vi "b2b2.vi"   [LabVIEW 2016, in "Moving Motor.lvrbt"]
uses:
  Moving Motor.lvrbt
  <vilib>/NXT/Block Support/NXT_InputPort.ctl
  <vilib>/NXT/Hardware/Plugins/Tetrix 180 deg Servo/Tetrix180ServoAddress.ctl
  <vilib>/NXT/Hardware/Plugins/Tetrix DC Motor/TetrixDCMotorAddress.ctl
  <vilib>/NXT/NXTIO Xnodes/NXTIONodeSubVIs/TETRIX IO Move Servos.vi
  <vilib>/NXT/NXTIO Xnodes/NXTIONodeSubVIs/TETRIX IO Move DC Motors.vi
  <vilib>/NXT/NXTIO Xnodes/NXTIONodeSubVIs/TETRIX IO Stop DC Motors.vi
  <vilib>/NXT/Dual Mode Library/Sensors/EV3_Ultrasonic_CM.vi
  <vilib>/NXT/Dual Mode Library/Waits/Wait_EV3_Ultrasonic_Centimeter_Closer.vi
  <vilib>/NXT/NXTIO Xnodes/AddressXNode/NXTIOAddress.xnode
  <vilib>/NXT/Subs/LVHSConnector.ctl
  <vilib>/NXT/NXTIO Xnodes/NXTIOXNode/NXTIO.xnode
  <vilib>/NXT/LegoClasses/BrickReference/BrickReference.lvclass
types:
  T1 = typedef "NXT_InputPort.ctl" = u32
  T2 = typedef "Tetrix180ServoAddress.ctl" = i32
  T3 = cluster{"Tetrix180Servo":T2, "Tetrix180Servo":T2}
  T4 = typedef "LVHSConnector.ctl" = refnum<class "BrickReference.lvclass">
  T5 = typedef "TetrixDCMotorAddress.ctl" = i32
  T6 = cluster{"TetrixDCMotor":T5, "TetrixDCMotor 2":T5}
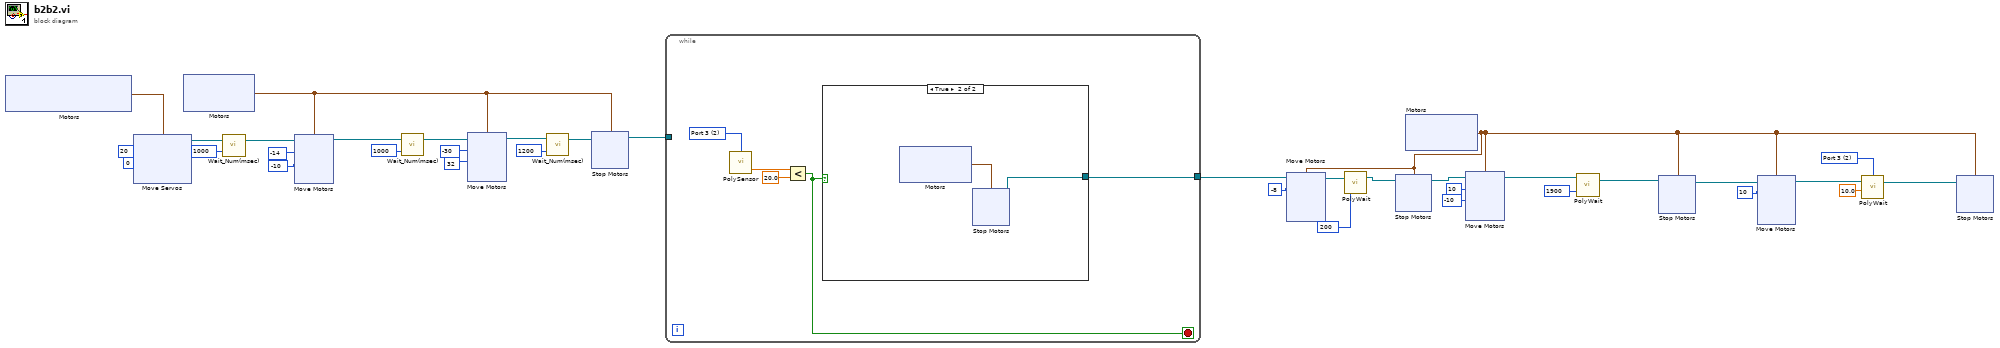
[diagram p0: block diagram]
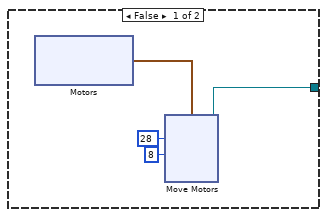
[diagram p2: hidden frame]
diagram:
  w7 = i8 -8 ("Power/Speed 1")
  w10 = T1 2 items=["Port 1", "Port 2", "Port 3", "Port 4"] ("Port (Port 1)")
  w12 = i8 10 ("Power/Speed 1")
  n1 = xnode "Motors"() -> ("Motor"=w35:T3)
  n2 = xnode "Move Servos"("Position 2"=u8 0, "Position 1"=u8 20, "Motors"=w35) -> ("NXT/EV3"=w32:T4)  [unwired: 1 in]
  n3 = xnode "Motors"() -> ("Motor"=w21:cluster{"TetrixDCMotor":T5, "TetrixDCMotor":T5})
  n4 = call <vilib>:"Wait_Num(msec).vi"("Time (100 msec)"=u32 1000, "NXT/EV3"=w32) -> ("NXT/EV3"=w31:T4)  [unwired: 2 in]
  n5 = xnode "Move Motors"("Power/Speed 2"=i8 -10, "Power/Speed 1"=i8 -14, "Motors"=w21, "NXT/EV3"=w31) -> ("NXT/EV3"=w27:T4)
  n6 = call <vilib>:"Wait_Num(msec).vi"("Time (100 msec)"=u32 1000, "NXT/EV3"=w27) -> ("NXT/EV3"=w20:T4)  [unwired: 2 in]
  n7 = xnode "Move Motors"("Power/Speed 2"=i8 32, "Power/Speed 1"=i8 -30, "Motors"=w21, "NXT/EV3"=w20) -> ("NXT/EV3"=w23:T4)
  n8 = call <vilib>:"Wait_Num(msec).vi"("Time (100 msec)"=u32 1200, "NXT/EV3"=w23) -> ("NXT/EV3"=w22:T4)  [unwired: 2 in]
  n9 = xnode "Stop Motors"("Motors"=w21, "NXT/EV3"=w22) -> ("NXT/EV3"=w19:T4)
  n10 = while {
    tunnel: w19 -> [_]
    tunnel: [w37] -> w6
    stop <- w38 stop-if-true
    w39 = T1 2 items=["Port 1", "Port 2", "Port 3", "Port 4"] ("Port (Port 1)")
    n11 = call-poly <vilib>:"PolySensor.vi"("Port (Port 1)"=w39) -> ("Centimeters"=w41:sgl)  [unwired: 2 in, 1 out]
    n12 = Less?(x=w41, y=sgl 20.0) -> (x < y?=w38:bool)
    n13 = case shown="True" w38 {
      tunnel: [w42 w55] -> w37
      frame False {
        n14 = xnode "Motors"() -> ("Motor"=w45:cluster{"TetrixDCMotor":T5, "TetrixDCMotor":T5})
        n15 = xnode "Move Motors"("Power/Speed 2"=i8 8, "Power/Speed 1"=i8 28, "Motors"=w45) -> ("NXT/EV3"=w42:T4)  [unwired: 1 in]
      }
      frame True {
        n16 = xnode "Motors"() -> ("Motor"=w56:cluster{"TetrixDCMotor":T5, "TetrixDCMotor":T5})
        n17 = xnode "Stop Motors"("Motors"=w56) -> ("NXT/EV3"=w55:T4)  [unwired: 1 in]
      }
    }
  }
  n18 = xnode "Motors"() -> ("Motor"=w3:cluster{"TetrixDCMotor":T5, "TetrixDCMotor":T5})
  n19 = xnode "Move Motors"("Power/Speed 2"=w7, "Power/Speed 1"=w7, "Motors"=w3, "NXT/EV3"=w6) -> ("NXT/EV3"=w5:T4)
  n20 = call-poly <vilib>:"PolyWait.vi"("Time (100 msec)"=u32 200, "NXT/EV3"=w5) -> ("NXT/EV3"=w2:T4)  [unwired: 2 in]
  n21 = xnode "Stop Motors"("Motors"=w3, "NXT/EV3"=w2) -> ("NXT/EV3"=w1:T4)
  n22 = xnode "Move Motors"("Power/Speed 2"=i8 -10, "Power/Speed 1"=i8 10, "Motors"=w3, "NXT/EV3"=w1) -> ("NXT/EV3"=w16:T4)
  n23 = call-poly <vilib>:"PolyWait.vi"("Time (100 msec)"=u32 1900, "NXT/EV3"=w16) -> ("NXT/EV3"=w14:T4)  [unwired: 2 in]
  n24 = xnode "Stop Motors"("Motors"=w3, "NXT/EV3"=w14) -> ("NXT/EV3"=w13:T4)
  n25 = xnode "Move Motors"("Power/Speed 2"=w12, "Power/Speed 1"=w12, "Motors"=w3, "NXT/EV3"=w13) -> ("NXT/EV3"=w11:T4)
  n26 = call-poly <vilib>:"PolyWait.vi"("Centimeters (40)"=sgl 10.0, "NXT/EV3"=w11, "Port (Port 1)"=w10) -> ("NXT/EV3"=w8:T4)  [unwired: 1 in]
  n27 = xnode "Stop Motors"("Motors"=w3, "NXT/EV3"=w8) -> ()  [unwired: 1 out]
